vi "dfd_Get Structure Property Id.vi"(0 "structure type":T3) -> (1 "filter structure id":T2, 2 "filter structure form id":T1)   [LabVIEW 2017, in "NI_DigFilterLicensed.lvlib"]
uses:
  <vilib>/addons/Digital Filter Design/NI_DigFilterLicensed.lvlib
  <vilib>/addons/Digital Filter Design/_Objects.llb/DFD Filter Structure Type Selector.ctl
  <vilib>/addons/Digital Filter Design/_Objects.llb/DFD Filter Structure Id.ctl
  <vilib>/addons/Digital Filter Design/_Objects.llb/DFD Filter Structure Form Id.ctl
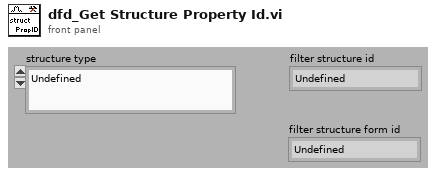
[diagram p1: front panel]
types:
  T1 = typedef "NI_DigFilterLicensed.lvlib/DFD Filter Structure Form Id.ctl" = enum16{"Undefined", "Direct Form", "SOS Form", "Lattice Form"}
  T2 = typedef "NI_DigFilterLicensed.lvlib/DFD Filter Structure Id.ctl" = enum16{"Undefined", "FIR", "IIR Direct", "IIR SOS", "IIR Allpass", "IIR AR", "IIR ARMA"}
  T3 = typedef "NI_DigFilterLicensed.lvlib/DFD Filter Structure Type Selector.ctl" = enum16{"Undefined", "FIR Direct Form", "FIR Direct Form Transposed", "FIR Symmetric", "FIR Antisymmetric", "IIR Direct Form I", "IIR Direct Form I Transposed", "IIR Direct Form II", "IIR Direct Form II Transposed", "IIR Cascaded Second Order Sections Form I", "IIR Cascaded Second Order Sections Form I Transposed", "IIR Cascaded Second Order Sections Form II", "IIR Cascaded Second Order Sections Form II Transposed", "Lattice Allpass (basic sections)", "Lattice Allpass (one multiplier sections)", "Lattice Allpass (normalized sections)", "Lattice AR (basic sections)", "Lattice AR (one multiplier sections)", "Lattice AR (normalized sections)", "Lattice MA (minimum phase)", "Lattice MA (maximum phase)", "Lattice ARMA (basic sections)", "Lattice ARMA (one multiplier sections)", "Lattice ARMA (normalized sections)"}
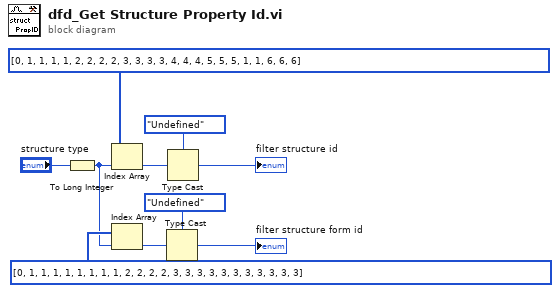
[diagram p0: block diagram]
diagram:
  n1 = To Long Integer(number="structure type") -> (32bit integer=w4:i32)
  n2 = Index Array(array=u16[] [0, 1, 1, 1, 1, 2, 2, 2, 2, 3, 3, 3, 3, 4, 4, 4, 5, 5, 5, 1, 1, 6, 6, 6], index=w4) -> (element=w9:u16)
  n3 = Index Array(array=u16[] [0, 1, 1, 1, 1, 1, 1, 1, 1, 2, 2, 2, 2, 3, 3, 3, 3, 3, 3, 3, 3, 3, 3, 3], index=w4) -> (element=w3:u16)
  n4 = Type Cast(type=DFD_Filter_Structure_Form_Id."Undefined" ("filter structure form id"), x=w3) -> (*(type *) &x=→"filter structure form id":T1)
  n5 = Type Cast(type=DFD_Filter_Structure_Id."Undefined" ("filter structure id"), x=w9) -> (*(type *) &x=→"filter structure id":T2)
